vi "SerialPort.Config_All.vi"(6 "Timeout ms (3sec)":u32=3000, 7 "State Ctrl Ref":refnum<vi>, 8 "error in (no error)":errorcluster, 9 "Config":T1={"Baud Rate (115200)"=115200, "Data Bits (8)"=8, "Parity (0:none)"=enum."None", "Stop Bits (10: 1 bit)"=10, "Flow Control (0:none)"=enum."None", "Enable Term Char (T)"=TRUE, "Term Char(0xA = '\\n' = LF) "=10} {"Term Char(0xA = '\\n' = LF)" format="%.0x"; "Stop Bits (10: 1 bit)" items=["1.0"=10, "1.5"=15, "2.0"=20]; "Data Bits (8)" min=5 max=8 step=1}, 10 "Com Port":refnum<visa-resource-name>="COM3", 11 "SerialPort in":refnum<class "SerialPort.lvclass">) -> (0 "error out":errorcluster, 3 "SerialPort out":refnum<class "SerialPort.lvclass">)   [LabVIEW 2018, in "SerialPort.lvclass"]
uses:
  SerialPort.lvclass
  Controls/SeroalPort.Config Settings.ctl
  Controls/SerialPort.Status Enum.ctl
  SerialPort.lvclass/SerialPort.ctl
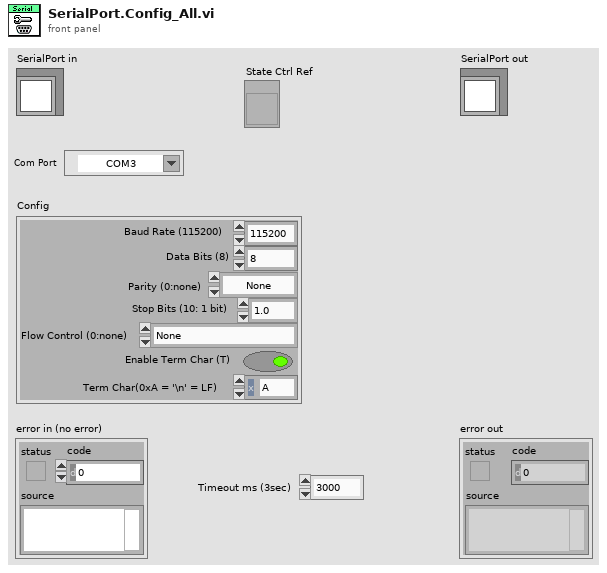
[diagram p1: front panel]
types:
  T1 = typedef "SeroalPort.Config Settings.ctl" = cluster{"Baud Rate (115200)":u32, "Data Bits (8)":u16, "Parity (0:none)":enum16{"None", "Odd", "Even", "Mark", "Space"}, "Stop Bits (10: 1 bit)":u16, "Flow Control (0:none)":enum16{"None", "XON/XOFF", "RTS/CTS", "XON/XOFF & RTS/CTS", "DTR/DSR", "XON/XOFF & DTR/DSR"}, "Enable Term Char (T)":bool, "Term Char(0xA = '\\n' = LF) ":u8}
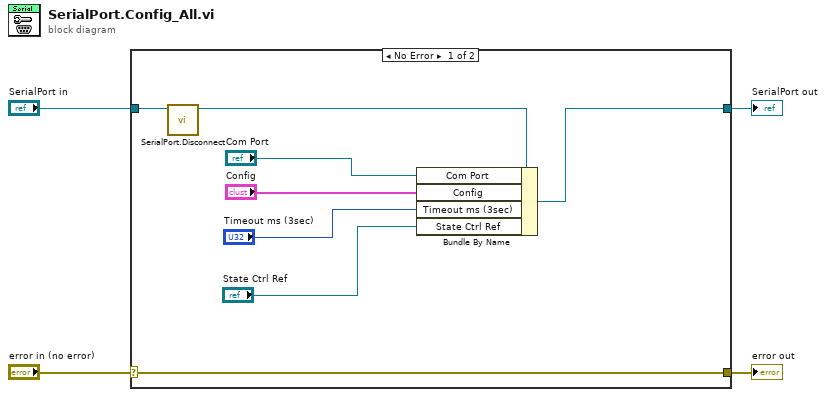
[diagram p0: block diagram]
diagram:
  n1 = case shown="No Error" "error in (no error)" {
    selector: "error in (no error)" -> [w12 w14]
    tunnel: [w12 w14] -> w3
    tunnel: [w5 w13] -> w1
    tunnel: "SerialPort in" -> [w7 w13]
    frame No Error {
      n2 = call "SerialPort.Disconnect.vi"("SerialPort in"=w7) -> ("SerialPort out"=w6:refnum<class "SerialPort.lvclass">)  [unwired: 8 in, 2 out]
      n3 = Bundle By Name(cluster=w6, "Com Port"="Com Port", "Config"="Config", "Timeout ms (3sec)"="Timeout ms (3sec)", "State Ctrl Ref"="State Ctrl Ref") -> (w5:refnum<class "SerialPort.lvclass">)
    }
    frame Error {
    }
  }
  "error out" <- w3
  "SerialPort out" <- w1
